vi "destroyPubDataEvents.vi"(8 "error in (no error)":errorcluster, 11 "UserEvents in":refnum<class "UserEvents.lvclass">) -> (0 "error out":errorcluster, 3 "UserEvents out":refnum<class "UserEvents.lvclass">)   [LabVIEW 2013, in "UserEvents.lvclass"]
uses:
  UserEvents.lvclass
  UserEvents.lvclass/UserEvents.ctl
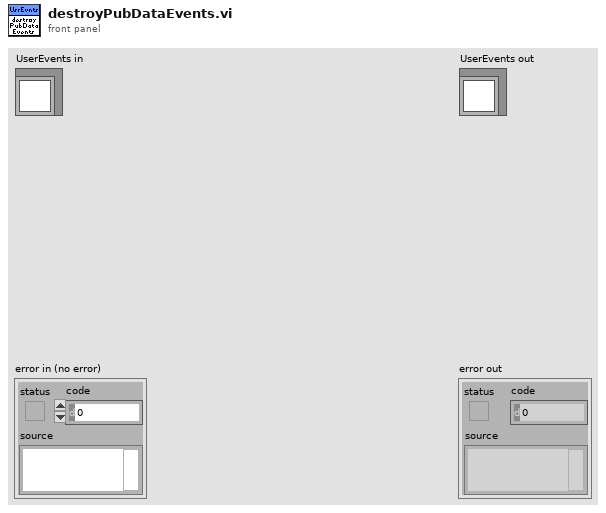
[diagram p1: front panel]
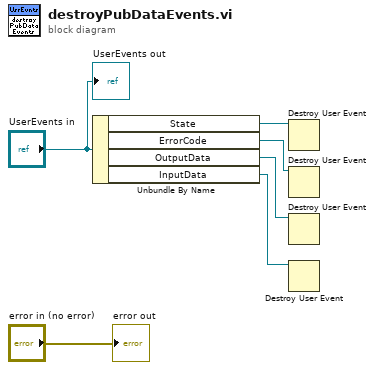
[diagram p0: block diagram]
diagram:
  n1 = Unbundle By Name("UserEvents in") -> ("State"=w5:refnum<user-event>, "ErrorCode"=w4:refnum<user-event>, "OutputData"=w3:refnum<user-event>, "InputData"=w2:refnum<user-event>)
  n2 = Destroy User Event(user event=w5) -> ()  [unwired: 1 in, 1 out]
  n3 = Destroy User Event(user event=w4) -> ()  [unwired: 1 in, 1 out]
  n4 = Destroy User Event(user event=w3) -> ()  [unwired: 1 in, 1 out]
  n5 = Destroy User Event(user event=w2) -> ()  [unwired: 1 in, 1 out]
  "error out" <- "error in (no error)"
  "UserEvents out" <- "UserEvents in"
